vi "BayesianRegressors.vi"   [LabVIEW 2020]
doc: "Polymorphic VI for bayesian regressors"
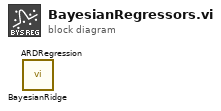
[diagram p0: block diagram]
diagram:
  n1 = call "BayesianRidge.vi"() -> ()  [unwired: 10 in, 2 out]
  n2 = call "ARDRegression.vi"() -> ()  [unwired: 10 in, 2 out]
